vi "LookUpChannel.vi"(8 "error in (no error)":errorcluster, 11 "Parameters":string="deviceid=0x35089") -> (0 "error out":errorcluster, 2 "FoundChannel out":u16 format="%.0x", 3 "Parameters out":string)   [LabVIEW 2023, in "PCAN API.lvlib"]
doc: "This VI is used to find port connected to a defined parameter. \nHere it is used for finding number of port connected to defined ID (deviceid=0x35089)"
uses:
  PCAN API.lvlib
  PCAN2023/PCAN2023.lvlib
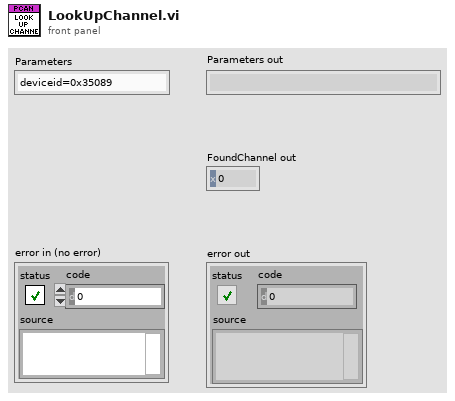
[diagram p1: front panel]
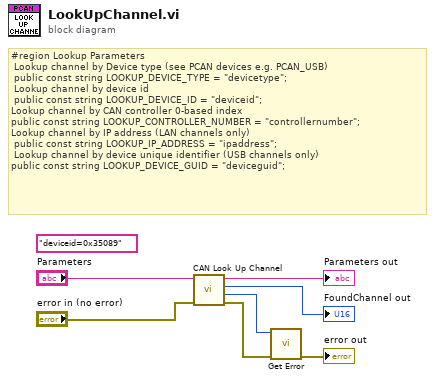
[diagram p0: block diagram]
diagram:
  (unwired) "deviceid=0x35089" ("Parameters")
  # "#region Lookup Parameters\n Lookup channel by Device type (see PCAN devices e.g. PCAN_USB)\n public const string LOOKUP_DEVICE_TYPE = \"devicetype\";\n Lookup channel by device id\n public const string LOOKUP_DEVICE_ID = \"deviceid\";\nLookup channel by CAN controller 0-based index\npublic const string LOOKUP_CONTROLLER_NUMBER = \"controllernumber\";\nLookup channel by IP address (LAN channels only)\n public const string LOOKUP_IP_ADDRESS = \"ipaddress\";\n Lookup channel by device unique identifier (USB channels only)\npublic const string LOOKUP_DEVICE_GUID = \"deviceguid\";"
  n1 = call "CAN Look Up Channel.vi"("error in (no error)"="error in (no error)", "Parameters"="Parameters") -> ("error out"=w2:errorcluster, "function return"=w4:u32, "FoundChannel out"=→"FoundChannel out":u16, "Parameters out"=→"Parameters out":string)  [unwired: 6 in]
  n2 = call "Get Error.vi"("error in (no error)"=w2, "function return"=w4) -> ("error out"=→"error out":errorcluster)  [unwired: 9 in]
